vi "Get User Info.vi"(8 "error in":errorcluster) -> (0 "error out":errorcluster, 1 "User Name":string, 2 "User Domain":string, 3 "Computer Name":string, 4 "Domain Ext":string, 5 "Registered Owner":string, 6 "net address":u32, 7 "Registered Organization":string)   [LabVIEW 2018]
doc: "This VI retrieves user and computer network information."
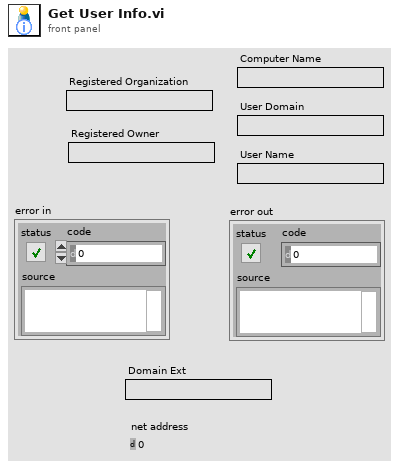
[diagram p1: front panel]
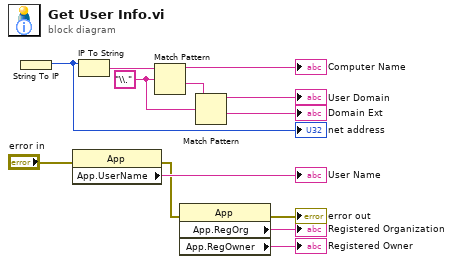
[diagram p0: block diagram]
diagram:
  w8 = "\\." ("regular expression")
  n1 = String To IP() -> (0:w11:u32)  [unwired: 1 in]
  "net address" <- w11
  n2 = property class="App"(error in="error in") -> (error out=w3:errorcluster, "App.UserName"=→"User Name":string)  [unwired: 1 in, 1 out]
  n3 = IP To String(2:w11) -> (0:w10:string)  [unwired: 1 in]
  n4 = Match Pattern(string=w10, regular expression=w8) -> (before substring=→"Computer Name":string, after substring=w9:string)  [unwired: 1 in, 2 out]
  n5 = property class="App"(error in=w3) -> (error out=→"error out":errorcluster, "App.RegOrg"=→"Registered Organization":string, "App.RegOwner"=→"Registered Owner":string)  [unwired: 1 in, 1 out]
  n6 = Match Pattern(string=w9, regular expression=w8) -> (before substring=→"User Domain":string, after substring=→"Domain Ext":string)  [unwired: 1 in, 2 out]
